vi "ssh2.vi"() -> ()   [LabVIEW 2017]
doc: "This VI illustrates how to connect to a remote SSH server."
uses:
  <vilib>/Utility/sysdir.llb/System Directory Type.ctl
  libssh2/libssh2_knownhost_typemask.ctl
  libssh2/libssh2_session_handshake_tcp.vi
  libssh2/libssh2_init_default.vi
  libssh2/libssh2_session_init_ex.vi
  <vilib>/Utility/tcp.llb/TCP Get Raw Net Object.vi
  libssh2/libssh2_session_handshake_socket.vi
  libssh2/libssh2_userauth_password_ex.vi
  libssh2/libssh2_channel_open_ex.vi
  libssh2/libssh2_channel_process_startup.vi
  libssh2/libssh2_channel_read_ex.vi
  libssh2/libssh2_session_disconnect_ex.vi
  libssh2/libssh2.lvlib
panel:
  out "exit status":i32
  in  "command":string="echo \"Hello World\""
  out "response":string
  in  "password":string
  in  "username":string
  in  "address":string
  out "error out":errorcluster
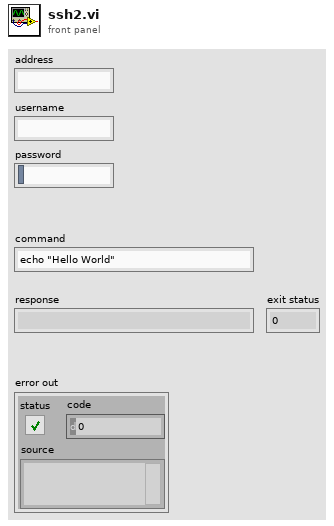
[diagram p1: front panel]
types:
  T1 = typedef "libssh2.lvlib/libssh2_knownhost_typemask.ctl" = i32
  T2 = typedef "System Directory Type.ctl" = i32
  T3 = typedef "libssh2.lvlib/Session Refnum.ctl" = refnum<k1>
  T4 = typedef "libssh2.lvlib/Host Key Database Refnum.ctl" = refnum<k1>
  T5 = typedef "libssh2.lvlib/Host Key Check Result.ctl" = enum16{"Match", "Mismatch", "Not Found", "Failure"}
  T6 = typedef "libssh2.lvlib/Host Key Refnum.ctl" = refnum<k1>
  T7 = typedef "libssh2.lvlib/Channel Refnum.ctl" = refnum<k1>
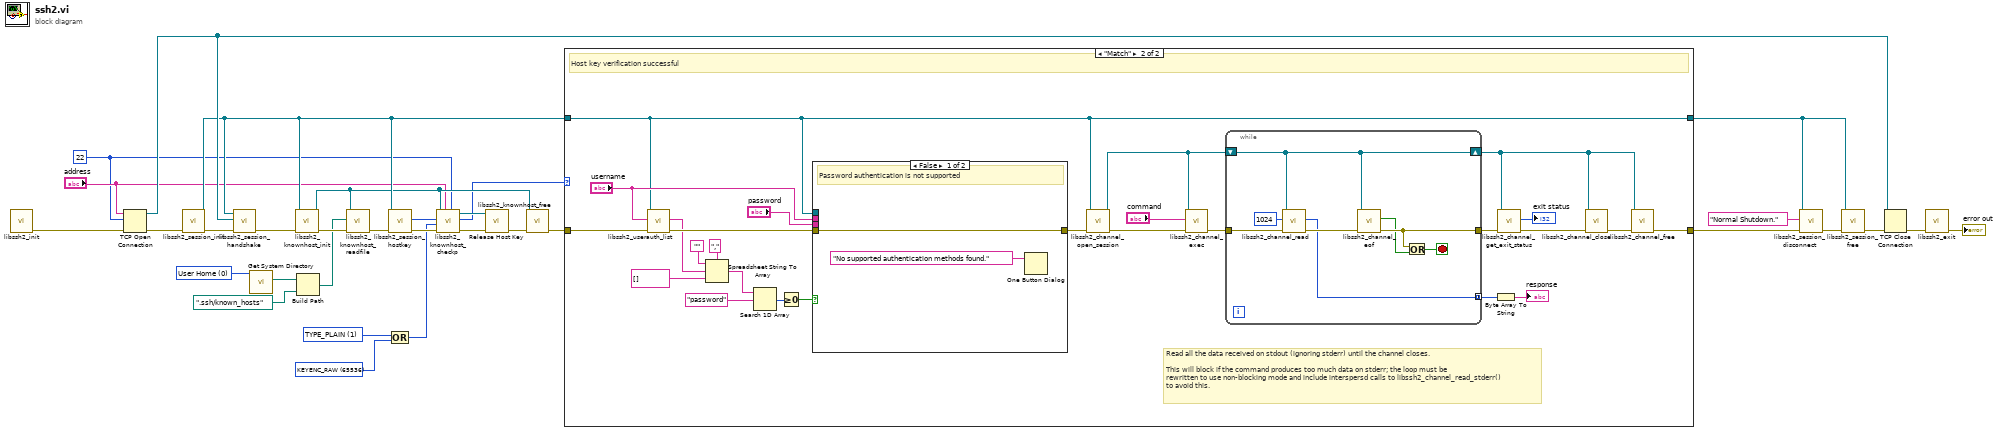
[diagram p0: block diagram]
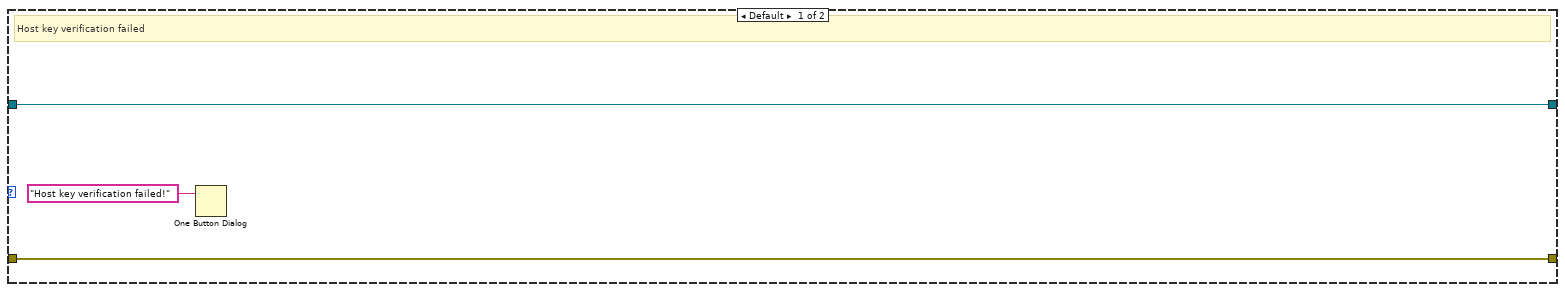
[diagram p2: hidden frame]
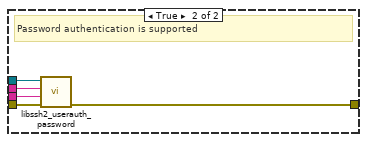
[diagram p3: hidden frame]
diagram:
  w2 = T1 65536 items=["TYPE_PLAIN"=1, "TYPE_SHA1"=2, "TYPE_CUSTOM"=3, "KEYENC_RAW"=65536, "KEYENC_BASE64"=131072, "KEY_RSA1"=262144, "KEY_SSHRSA"=524288, "KEY_SSHDSS (deprecated)"=786432, "KEY_ECDSA_256"=1048576, "KEY_ECDSA_384"=1310720, "KEY_ECDSA_521"=1572864, "KEY_ED25519"=1835008, "KEY_UNKNOWN"=3932160] ("typemask")
  w3 = T1 1 items=["TYPE_PLAIN"=1, "TYPE_SHA1"=2, "TYPE_CUSTOM"=3, "KEYENC_RAW"=65536, "KEYENC_BASE64"=131072, "KEY_RSA1"=262144, "KEY_SSHRSA"=524288, "KEY_SSHDSS (deprecated)"=786432, "KEY_ECDSA_256"=1048576, "KEY_ECDSA_384"=1310720, "KEY_ECDSA_521"=1572864, "KEY_ED25519"=1835008, "KEY_UNKNOWN"=3932160] ("typemask")
  w18 = T2 0 items=["User Home"=0, "User Desktop"=1, "User Documents"=2, "User Application Data"=3, "User Preferences"=4, "User Temporary"=5, "Public Documents"=6, "Public Application Data"=7, "Public Preferences"=8, "Public Cache"=13, "System Core Libraries"=9, "System Installed Libraries"=10, "Application Files"=11, "Boot Volume Root"=12] ("system directory type")
  w10 = u16 22 ("remote port or service name")
  n1 = call-poly "libssh2_init.vi"() -> ("error out"=w32:errorcluster)  [unwired: 11 in]
  n2 = TCP Open Connection(address="address", remote port or service name=w10, error in (no error)=w32) -> (connection ID=w23:refnum<k5>, error out=w24:errorcluster)  [unwired: 2 in]
  n3 = call "libssh2_session_init.vi"("error in (no error)"=w24) -> ("error out"=w29:errorcluster, "session"=w22:T3)  [unwired: 9 in]
  n4 = call-poly "libssh2_session_handshake.vi"("error in (no error)"=w29, "tcp connection"=w23, "session"=w22) -> ("error out"=w19:errorcluster)  [unwired: 8 in]
  n5 = call <vilib>:"Get System Directory.vi"("system directory type"=w18) -> ("system directory"=w17:path)  [unwired: 10 in]
  n6 = call "libssh2_knownhost_init.vi"("error in (no error)"=w19, "session"=w22) -> ("error out"=w15:errorcluster, "host key database"=w13:T4)  [unwired: 8 in]
  n7 = Build Path(base path=w17, name or relative path=path ".ssh/known_hosts") -> (appended path=w12:path)
  n8 = call "libssh2_knownhost_readfile.vi"("error in (no error)"=w15, "filename"=w12, "host key database"=w13) -> ("error out"=w14:errorcluster)  [unwired: 7 in, 1 out]
  n9 = call "libssh2_session_hostkey.vi"("error in (no error)"=w14, "session"=w22) -> ("error out"=w4:errorcluster, "hostkey"=w20:u8[])  [unwired: 7 in, 1 out]
  n10 = Compound Arithmetic op=OR(w3, w2) -> (w1:T1)
  n11 = call "libssh2_knownhost_checkp.vi"("port"=w10, "host"="address", "error in (no error)"=w4, "typemask"=w1, "key"=w20, "host key database"=w13) -> ("error out"=w8:errorcluster, "result"=w5:T5, "host key"=w6:T6)  [unwired: 3 in]
  n12 = call "Release Host Key.vi"("error in (no error)"=w8, "host key"=w6) -> ("error out"=w7:errorcluster)  [unwired: 9 in]
  n13 = call "libssh2_knownhost_free.vi"("error in (no error)"=w7, "host key database"=w13) -> ("error out"=w21:errorcluster)  [unwired: 9 in]
  n14 = case shown="\"Match\"" w5 {
    tunnel: [w34 w46] -> w27
    tunnel: w22 -> [w35 w36]
    tunnel: w21 -> [w34 w37]
    tunnel: [w35 w36] -> w9
    frame Default {
      # "Host key verification failed"
      n15 = One Button Dialog(message="Host key verification failed!") -> ()  [unwired: 1 in, 1 out]
    }
    frame "Match" {
      # "Read all the data received on stdout (ignoring stderr) until the channel closes.\n\nThis will block if the command produces too much data on stderr; the loop must be\nrewritten to use non-blocking mode and include interspersd calls to libssh2_channel_read_stderr()\nto avoid this."
      # "Host key verification successful"
      n16 = call "libssh2_userauth_list.vi"("error in (no error)"=w37, "username"="username", "session"=w36) -> ("error out"=w61:errorcluster, "supported authentication schemes"=w60:string)  [unwired: 7 in]
      n17 = Spreadsheet String To Array(delimiter (Tab)=",", format string="", spreadsheet string=w60, array type (2D Dbl)=string[] []) -> (array=w56:string[])
      n18 = Search 1D Array(1D array=w56, element="password") -> (index of element=w51:i32)  [unwired: 1 in]
      n19 = Greater Or Equal To 0?(x=w51) -> (x >= 0?=w50:bool)
      n20 = case shown="False" w50 {
        tunnel: w61 -> [w63 w68]
        tunnel: [w63 w67] -> w54
        tunnel: w36 -> [_ w66]
        tunnel: "username" -> [_ w65]
        tunnel: "password" -> [_ w64]
        frame False {
          # "Password authentication is not supported"
          n21 = One Button Dialog(message="No supported authentication methods found.") -> ()  [unwired: 1 in, 1 out]
        }
        frame True {
          # "Password authentication is supported"
          n22 = call "libssh2_userauth_password.vi"("error in (no error)"=w68, "password"=w64, "username"=w65, "session"=w66) -> ("error out"=w67:errorcluster)  [unwired: 7 in]
        }
      }
      n23 = call "libssh2_channel_open_session.vi"("error in (no error)"=w54, "session"=w36) -> ("error out"=w49:errorcluster, "channel"=w44:T7)  [unwired: 8 in]
      n24 = call "libssh2_channel_exec.vi"("error in (no error)"=w49, "command"="command", "channel"=w44) -> ("error out"=w48:errorcluster)  [unwired: 8 in]
      n25 = while {
        tunnel: w48 -> [w76]
        tunnel: [w74] -> w45
        shift-right: [w72] -> w39
        shift-left: w44 -> [w72]
        tunnel: [w70] -> w43 mode=concatenating
        stop <- w75 stop-if-true
        n26 = call "libssh2_channel_read.vi"("error in (no error)"=w76, "buffer length"=i64 1024 ("buflen"), "channel"=w72) -> ("error out"=w73:errorcluster, "buffer"=w70:u8[])  [unwired: 7 in]
        n27 = call "libssh2_channel_eof.vi"("error in (no error)"=w73, "channel"=w72) -> ("error out"=w74:errorcluster, "eof"=w69:bool)  [unwired: 8 in]
        n28 = Or(x=w74, y=w69) -> (x .or. y?=w75:bool)
      }
      n29 = Byte Array To String(unsigned byte array=w43) -> (string=→"response":string)
      n30 = call "libssh2_channel_get_exit_status.vi"("error in (no error)"=w45, "channel"=w39) -> ("error out"=w41:errorcluster, "exit status"=→"exit status":i32)  [unwired: 8 in]
      n31 = call "libssh2_channel_close.vi"("error in (no error)"=w41, "channel"=w39) -> ("error out"=w40:errorcluster)  [unwired: 9 in]
      n32 = call "libssh2_channel_free.vi"("error in (no error)"=w40, "channel"=w39) -> ("error out"=w46:errorcluster)  [unwired: 9 in]
    }
  }
  n33 = call "libssh2_session_disconnect.vi"("error in (no error)"=w27, "description"="Normal Shutdown.", "session"=w9) -> ("error out"=w26:errorcluster)  [unwired: 8 in]
  n34 = call "libssh2_session_free.vi"("error in (no error)"=w26, "session"=w9) -> ("error out"=w28:errorcluster)  [unwired: 9 in]
  n35 = TCP Close Connection(connection ID=w23, error in (no error)=w28) -> (error out=w30:errorcluster)  [unwired: 1 in, 1 out]
  n36 = call "libssh2_exit.vi"("error in (no error)"=w30) -> ("error out"=→"error out":errorcluster)  [unwired: 10 in]
